vi "SOUR_POW_COUP_ON_OFF.vi"(0 "VISA IN":refnum<visa-resource-name>, 1 "Coupling ON/OFF":bool, 5 "error in":errorcluster, 7 "Channel":i32) -> (14 "VISA Out":refnum<visa-resource-name>, 19 "error out":errorcluster)   [LabVIEW 2018, in "PNA-X.lvlib"]
doc: "SOURce<cnum>:POWer:COUPle <ON | OFF> \n(Read-Write) Turns Port Power Coupling ON or OFF. \nParameters \n<cnum> Any existing channel number. If unspecified, value is set to 1 \n<ON | OFF> ON (or 1) - turns coupling ON. The same power level is used for both source \nports. \nOFF (or 0) - turns coupling OFF. Power level can be set individually for each \nsource port. \nExamples SOUR:POW:COUP ON \nsource2:power:couple off \nQuery Syntax SOURce<cnum>:POWer:COUPle? \nReturn Type Boolean (1 = ON, 0 = OFF) \nDefault ON"
uses:
  PNA-X.lvlib
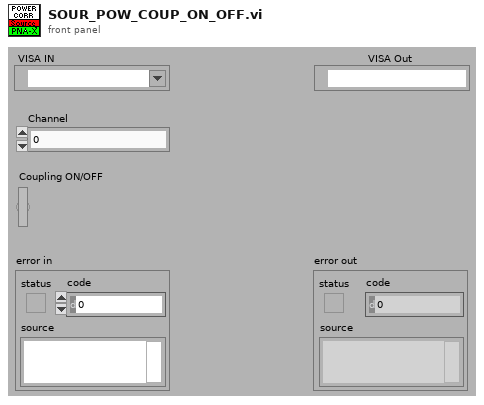
[diagram p1: front panel]
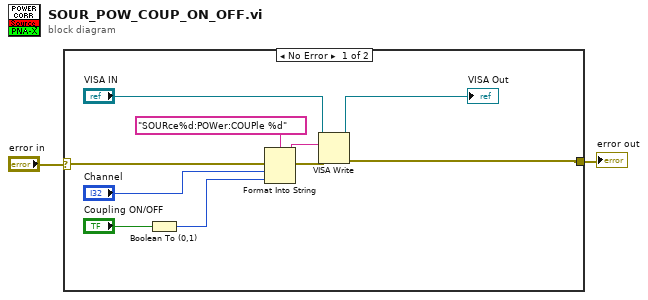
[diagram p0: block diagram]
diagram:
  n1 = case shown="No Error" "error in" {
    selector: "error in" -> [w12 w13]
    tunnel: [w7 w13] -> w1
    frame No Error {
      n2 = Boolean To (0,1)(Boolean="Coupling ON/OFF") -> (0, 1=w3:i16)
      n3 = Format Into String(format string="SOURce%d:POWer:COUPle %d" ("Cmdline"), error in=w12, "Channel", w3) -> (resulting string=w10:string, error out=w11:errorcluster)  [unwired: 1 in]
      n4 = VISA Write(VISA resource name="VISA IN", write buffer=w10, error in (no error)=w11) -> (VISA resource name out=→"VISA Out":refnum<visa-resource-name>, error out=w7:errorcluster)  [unwired: 1 out]
    }
    frame Error {
    }
  }
  "error out" <- w1
